vi "readStickEnc.vi"(6 "Reset Counter":bool, 7 "Reverse ENC?":bool, 8 "error in (no error)":errorcluster) -> (0 "error out":errorcluster, 2 "StickEncoder (deg)":dbl)   [LabVIEW 2019, in "SJCube.lvlib"]
uses:
  SJCube.lvlib
  <vilib>/myRIO/Common/Instrument Driver Framework/myRIO v1.0/Encoder/typedefs/Encoder Count Direction Enum.ctl
  <vilib>/myRIO/Common/Instrument Driver Framework/myRIO v1.0/Encoder/typedefs/Encoder Signal Mode.ctl
  <vilib>/myRIO/Common/Instrument Driver Framework/myRIO v1.0/Encoder/typedefs/Encoder Channels Enum.ctl
  <vilib>/myRIO/Common/Instrument Driver Framework/Utilities/typedefs/Generic FPGA Reference.ctl
  <vilib>/myRIO/Common/Instrument Driver Framework/Utilities/typedefs/myRIO v1.0 Reference.ctl
  <vilib>/myRIO/Common/Instrument Driver Framework/Utilities/typedefs/Hardware Version Enum.ctl
  <vilib>/myRIO/Common/Instrument Driver Framework/Utilities/typedefs/myRIO Generic Hardware Reference.ctl
  <vilib>/myRIO/Instrument Drivers/Onboard IO/Encoder/typedefs/Encoder Reference.ctl
  <vilib>/myRIO/Instrument Drivers/Onboard IO/Encoder/Encoder.lvlib
  <vilib>/myRIO/Instrument Drivers/Onboard IO/Encoder/vis/Read.vi
  <vilib>/myRIO/Instrument Drivers/Onboard IO/Encoder/vis/myRIO Encoder Open.xnode
  <vilib>/myRIO/Common/Instrument Driver Framework/Utilities/vis/Is FPGA Ref Available.vi
  <vilib>/myRIO/Express VI/Onboard IO/Encoder/Encoder Express VI.xnode
  <vilib>/myRIO/Common/Instrument Driver Framework/myRIO v1.0/Encoder/vis/myRIO v1.0 Configure Encoder.vi
  <vilib>/myRIO/Common/Instrument Driver Framework/myRIO v1.0/Encoder/typedefs/Encoder Configuration v1.0.ctl
  <vilib>/userDefined/High Color/nirio_resource_hc.ctl
  KNRmBalanceStick-Program/KNRm_ReMi_OS5.lvlibp/KNRm_ReMi_Toolkit/IO/LowLevel/IO_Channel_Motor.ctl
  <vilib>/myRIO/Common/Instrument Driver Framework/myRIO v1.0/Encoder/vis/myRIO v1.1 Open Encoder.vi
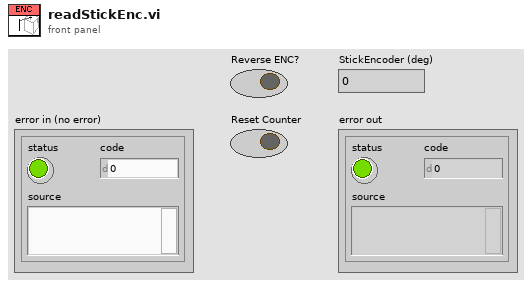
[diagram p1: front panel]
types:
  T1 = typedef "KNRm_ReMi_OS5.lvlibp/IO_Channel_Motor.ctl" = enum16{"M1", "M2", "M3", "M4"}
  T2 = typedef "Encoder.lvlib/Encoder Reference.ctl" = cluster{"myRIO Reference":T3, "Encoder Channels Enum":T7}
  T3 = typedef "myRIO Generic Hardware Reference.ctl" = cluster{"myRIO Model":T4, "myRIO Hardware Reference":T5}
  T4 = typedef "Hardware Version Enum.ctl" = enum16{"Unknown", "myRIO-1900", "myRIO-1950", "roboRIO", "NI ELVIS RIO CM", "ELVIS III"}
  T5 = typedef "myRIO v1.0 Reference.ctl" = cluster{"Generic FPGA Reference":T6, "Allow multiple opens":bool}
  T6 = typedef "Generic FPGA Reference.ctl" = refnum<k20>
  T7 = typedef "Encoder Channels Enum.ctl" = enum16{"Not Connected", "C/ENC0", "C/ENC1", "A/ENC", "A/ENC0", "A/ENC1", "A/ENC2", "A/ENC3", "A/ENC4", "A/ENC5", "A/ENC6", "A/ENC7", "A/ENC8", "A/ENC9", "B/ENC", "B/ENC0", "B/ENC1", "B/ENC2", "B/ENC3", "B/ENC4", "B/ENC5", "B/ENC6", "B/ENC7", "B/ENC8", "B/ENC9", "DIO/ENC0", "DIO/ENC1", "DIO/ENC2", "DIO/ENC3", "DIO/ENC4"}
  T8 = typedef "Encoder Signal Mode.ctl" = enum16{"Quadrature phase signal", "Step and direction signal"}
  T9 = typedef "nirio_resource_hc.ctl" = tag
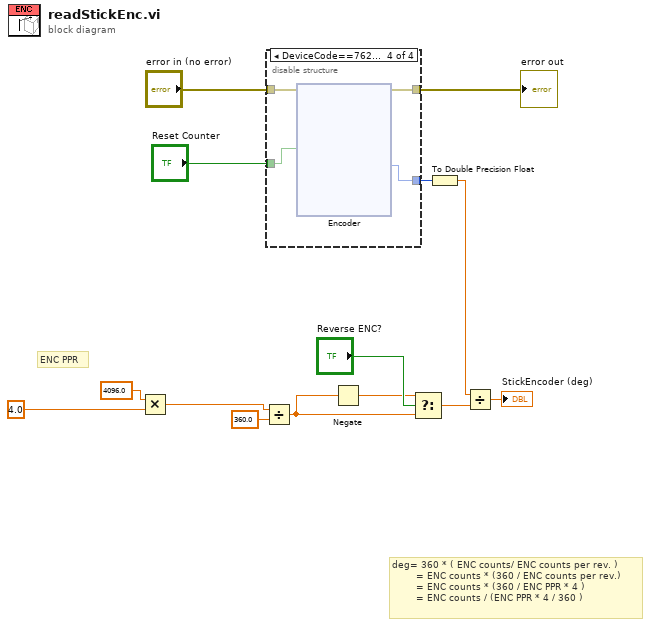
[diagram p0: block diagram]
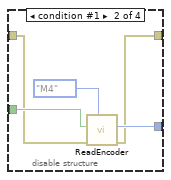
[diagram p3: hidden frame]
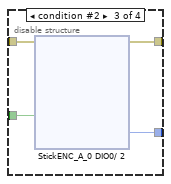
[diagram p4: hidden frame]
diagram:
  # "deg= 360 * ( ENC counts/ ENC counts per rev. )\n        = ENC counts * (360 / ENC counts per rev.)\n        = ENC counts * (360 / ENC PPR * 4 )\n        = ENC counts / (ENC PPR * 4 / 360 )"
  # "ENC PPR"
  n1 = Multiply(x=4096.0 ("y"), y=4.0) -> (x*y=w3:dbl)
  n2 = Divide(x=w3, y=360.0) -> (x/y=w1:dbl)
  n3 = disable-structure shown="DeviceCode==762F" {
    disable-tunnel: "error in (no error)" -> [w15 w17 w24 w74]
    disable-tunnel: [w15 w16 w21 w73] -> w9
    disable-tunnel: [_ w20 w22 w72] -> w8
    disable-tunnel: "Reset Counter" -> [_ w19 w23 w71]
    frame condition #0 (active) {
    }
    frame condition #1 {
      n4 = call "ReadEncoder.vi"("Channel"=IO_Channel_Motor."M4", "error in"=w17, "Reset"=w19) -> ("error out"=w16:errorcluster, "ENC (count)"=w20:i32)  [unwired: 7 in]
    }
    frame condition #2 {
      n5 = xnode "StickENC_A_0 DIO0/ 2"("Reset Counter"=w23, "error in (no error)"=w24) -> ("Counter Value"=w22:i32, "error out"=w21:errorcluster)  [unwired: 2 out]
    }
    frame condition #3 {
      n6 = xnode "Encoder"("Reset Counter"=w71, "error in (no error)"=w74) -> ("Counter Value"=w72:i32, "error out"=w73:errorcluster)  [unwired: 2 out]
    }
  }
  "error out" <- w9
  n7 = Negate(x=w1) -> (-x=w6:dbl)
  n8 = Select(t=w6, s="Reverse ENC?", f=w1) -> (s? t:f=w11:dbl)
  n9 = To Double Precision Float(number=w8) -> (double precision float=w13:dbl)
  n10 = Divide(x=w13, y=w11) -> (x/y=→"StickEncoder (deg)":dbl)
